vi "Copy of P3060_根据槽位打开设备.vi"(8 "error in (no error)":errorcluster caption="错误输入（无错误）", 10 "机箱号":i16=1, 11 "槽位号":i16) -> (0 "error out":errorcluster caption="错误输出", 3 "句柄输出":i32)   [LabVIEW 2010]
doc: "打开板卡操作，输出板卡句柄！当有多个板卡时，根据板卡索引号打开不同板卡！\n如果同时使用一块板卡的多种功能，可将输出句柄连接到不同的功能任务中。\n此VI是创建所有任务的前提！"
uses:
  _SubVI/dll/P3060.dll
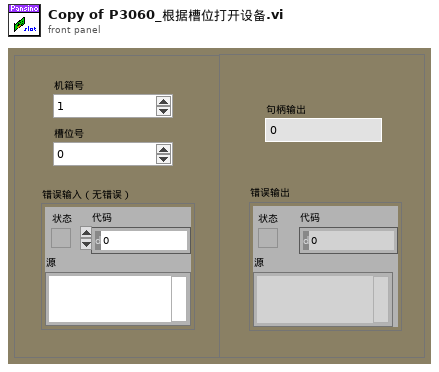
[diagram p1: front panel]
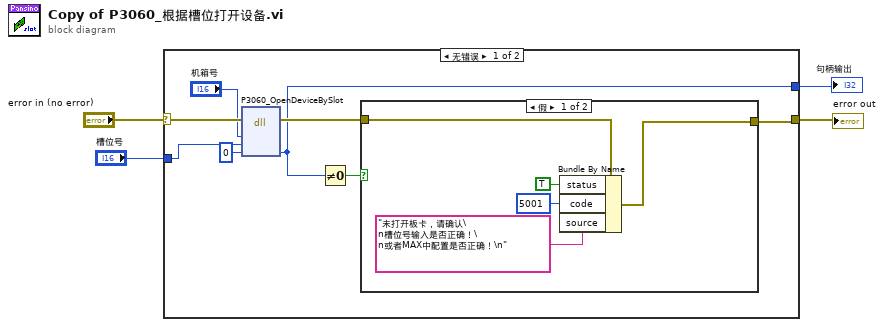
[diagram p0: block diagram]
diagram:
  n1 = case shown="无错误" "error in (no error)" {
    selector: "error in (no error)" -> [w12 w19]
    tunnel: [w8 w19] -> w1
    tunnel: "槽位号" -> [w11 _]
    tunnel: [w7 _] -> w3
    frame No Error {
      n2 = dll-call lib="D:/driver/trunk/Drivers/P3060/P3060API/P3060APILV/Labview/P3060/_SubVI/dll/P3060.dll" fn="P3060_OpenDeviceBySlot"(error in=w12, "Classis"="机箱号", "槽位号"=w11, "设备句柄"=0) -> (error out=w9:errorcluster, "设备句柄"=w7:i32)  [unwired: 5 in, 1 out]
      n3 = Not Equal To 0?(x=w7) -> (x != 0?=w10:bool)
      n4 = case shown="假" w10 {
        tunnel: w9 -> [w17 w18]
        tunnel: [w13 w18] -> w8
        frame False {
          n5 = Bundle By Name(cluster=w17, "status"=TRUE, "code"=5001, "source"="未打开板卡，请确认\n槽位号输入是否正确！\n或者MAX中配置是否正确！\n") -> (w13:errorcluster)
        }
        frame True {
        }
      }
    }
    frame Error {
    }
  }
  "句柄输出" <- w3
  "error out" <- w1
